vi "Set_integration_time.vi"(8 "error in":errorcluster, 11 "Integration Time":u8 format="%02x") -> (0 "error out":errorcluster)   [LabVIEW 2018]
panel:
  # "Integration time\nFF: 2.4ms\nF6: 10ms\nD5: 42ms\nC0: 64ms\n00: 700ms"
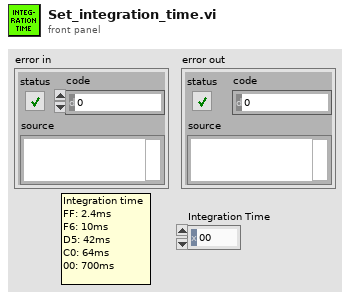
[diagram p1: front panel]
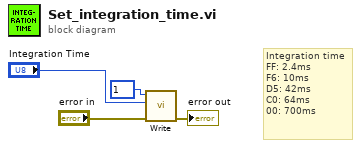
[diagram p0: block diagram]
diagram:
  # "Integration time\nFF: 2.4ms\nF6: 10ms\nD5: 42ms\nC0: 64ms\n00: 700ms"
  n1 = call "Write.vi"("error in"="error in", "Data to write"="Integration Time", "Address"=u8 1 ("Slave Address (7-bit)")) -> ("error out"=→"error out":errorcluster)  [unwired: 8 in]
